vi "习4.4.vi"() -> ()   [LabVIEW 2017]
panel:
  in  "数值":dbl
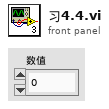
[diagram p1: front panel]
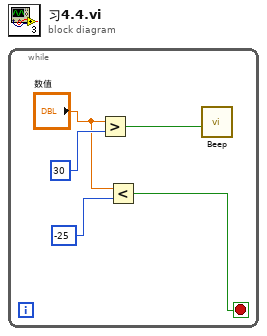
[diagram p0: block diagram]
diagram:
  n1 = while {
    stop <- w2 stop-if-true
    n2 = Greater?(x="数值", y=30) -> (0:w1:bool)
    n3 = Less?(x="数值", y=-25) -> (x < y?=w2:bool)
    n4 = call <vilib>:"Beep.vi"("use system alert? (T)"=w1) -> ()  [unwired: 11 in]
  }
